vi "Call NIPKG CLI.vi"(6 "custom configuration file path":path=path "", 8 "error in (no error)":errorcluster, 11 "command":string) -> (0 "error out":errorcluster, 3 "command line standard output":string)   [LabVIEW 2021, in "NIPM_API.lvlib"]
doc: "This VI calls the nipkg.exe command-line interface (CLI) from the command line.\n\nINPUT(s)\n<B>Command</B> is a string containing the specific nipkg CLI command (e.g. list-installed, feed-create, feed-add-pkg, etc) to execute.\n\nOUTPUT(s)\n<B>Command line standard output</B> returns the standard output information from the nipkg command that executed."
uses:
  NIPM_API.lvlib
panel:
  out "standard error":string
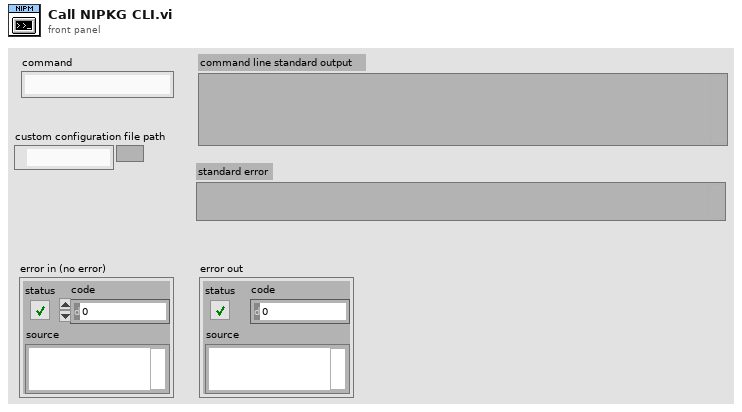
[diagram p1: front panel]
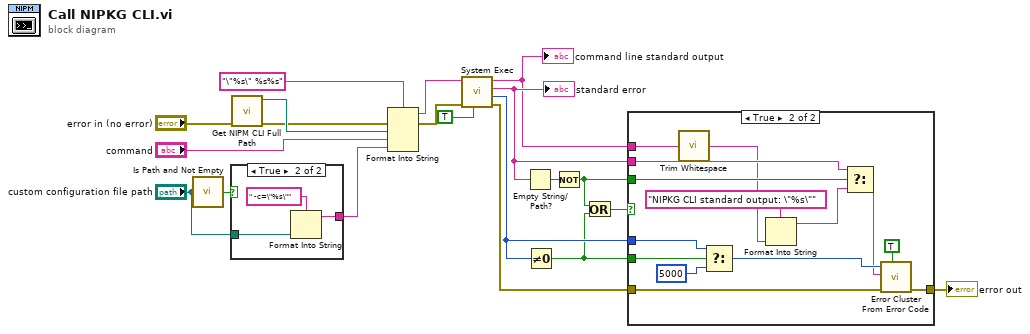
[diagram p0: block diagram]
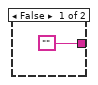
[diagram p2: hidden frame]
diagram:
  n1 = call <vilib>:"Is Path and Not Empty.vi"("path"="custom configuration file path") -> ("Is Path and Not Empty?"=w3:bool)  [unwired: 4 in]
  n2 = case shown="True" w3 {
    tunnel: "custom configuration file path" -> [_ w23]
    tunnel: ["" w22] -> w2
    frame False {
    }
    frame True {
      n3 = Format Into String(format string=" -c=\"%s\"", w23) -> (resulting string=w22:string)  [unwired: 2 in, 1 out]
    }
  }
  n4 = call "Get NIPM CLI Full Path.vi"("error in (no error)"="error in (no error)") -> ("error out"=w6:errorcluster, "NIPM CLI"=w8:path)  [unwired: 9 in]
  n5 = Format Into String(format string="\"%s\" %s%s", error in=w6, w8, "command", w2) -> (resulting string=w7:string, error out=w5:errorcluster)  [unwired: 1 in]
  n6 = call <vilib>:"System Exec.vi"("run minimized? (F)"=TRUE, "error in (no error)"=w5, "command line"=w7) -> ("error out"=w18:errorcluster, "return code"=w14:i32, "standard error"=w17:string, "standard output"=w11:string)  [unwired: 5 in]
  "command line standard output" <- w11
  "standard error" <- w17
  n7 = Empty String/Path?(string/path=w17) -> (empty?=w16:bool)
  n8 = Not Equal To 0?(x=w14) -> (x != 0?=w12:bool)
  n9 = Not(x=w16) -> (.not. x?=w13:bool)
  n10 = Or(x=w13, y=w12) -> (x .or. y?=w15:bool)
  n11 = case shown="True" w15 {
    tunnel: w18 -> [w25 w39]
    tunnel: w17 -> [_ w31]
    tunnel: [w25 w38] -> w19
    tunnel: w14 -> [_ w33]
    tunnel: w12 -> [_ w34]
    tunnel: w13 -> [_ w30]
    tunnel: w11 -> [_ w29]
    frame False {
    }
    frame True {
      n12 = call <vilib>:"Trim Whitespace.vi"("string"=w29) -> ("trimmed string"=w26:string)  [unwired: 1 in]
      n13 = Select(t=w33, s=w34, f=5000 ("error code (0)")) -> (s? t:f=w37:i32)
      n14 = Format Into String(format string="NIPKG CLI standard output: \"%s\"", w26) -> (resulting string=w27:string)  [unwired: 2 in, 1 out]
      n15 = Select(t=w31, s=w30, f=w27) -> (s? t:f=w35:string)
      n16 = call <vilib>:"Error Cluster From Error Code.vi"("show call chain? (False)"=TRUE, "error in (no error)"=w39, "error message (\"\")"=w35, "error code (0)"=w37) -> ("error out"=w38:errorcluster)  [unwired: 5 in]
    }
  }
  "error out" <- w19
